vi "16.扫描引擎同步高阶 (Host).vi"() -> ()   [LabVIEW 2019]
uses:
  <vilib>/Platform/TimedLoop/XDataNode/wakeup.ctl
  <vilib>/Platform/TimedLoop/XDataNode/XDNodeRunTimeDep.lvlib
  <vilib>/Platform/TimedLoop/XDataNode/nitl_modes.ctl
  <vilib>/Platform/TimedLoop/XDataNode/timing_clust.ctl
  <vilib>/Platform/TimedLoop/XDataNode/XDataNode.xnode
  <vilib>/rvi/interface/nirviReadWriteControl/nirviReadWriteControl.xnode
  <vilib>/rvi/interface/Simulation/niFpgaSimulationCallBeginRW.vi
  <vilib>/rvi/errors/niLvFpgaAdjustHostInterfaceError.vi
  <vilib>/rvi/interface/nirviCloseFPGA/nirviCloseFPGA.xnode
  <vilib>/rvi/interface/nirviOpenFPGA/nirviOpenFPGA.xnode
  <vilib>/Platform/TimedLoop/XDataNode/loadnilvce.vi
  <vilib>/FPGAPlugInAG/ELVIS III/niLvFpga_Open_ELVIS III.vi
  <vilib>/rvi/interface/common/dynamic/niFpgaDynamicAddResources.vi
  NiFpgaLv.dll
  <vilib>/Utility/error.llb/Error Cluster From Error Code.vi
  <vilib>/FPGAPlugInAG/Dynamic/niLvFpga_Close_Dynamic.vi
panel:
  out "Error Out":errorcluster
  in  "Reset Missed Falling Edge Latch":bool
  out "Missed Falling Edge Instantaneous":bool
  out "Scan Clock High Time (FPGA clock ticks)":u32
  in  "Adjust FPGA Acquisition Delay\n**Watch for Missed Falling Edge**":u32(slide) scale=0.0..1000000.0
  out "Missed Falling Edge Latched":bool
  out "Host Loop Finished Late? [i-1]":bool
  in  "stop":bool
  out "Digital Waveform Data from FPGA":i16(graph)
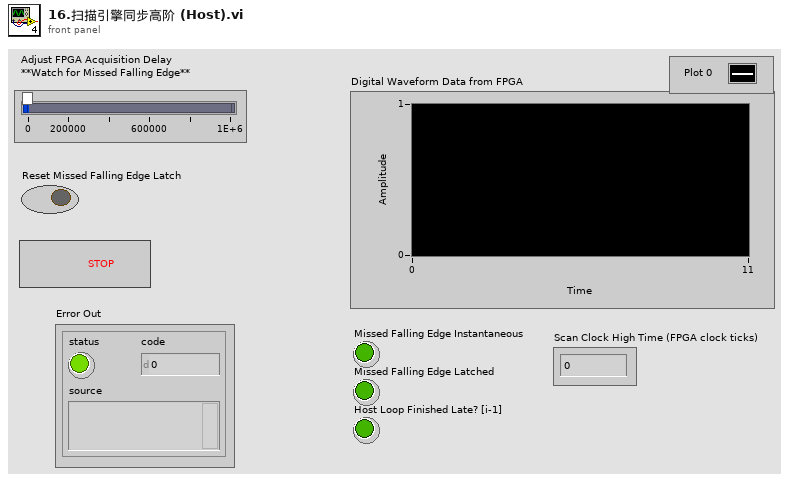
[diagram p1: front panel]
types:
  T1 = typedef "XDNodeRunTimeDep.lvlib/timing_clust.ctl" = cluster{"Expected End [f-1]":u64, "Actual End [f-1]":u64, "Finished Late? [f-1]":bool, "Expected End [i-1]":u64, "Actual End [i-1]":u64, "Finished Late? [i-1]":bool, "Expected Start [i]":u64, "Actual Start [i]":u64, "Expected Start [f]":u64, "Actual Start [f]":u64, "Source Name":string, "Structure Name":string, "Period":i64, "Deadline":i64, "Offset":i64, "Start":i64, "Priority":i32, "Timeout":i32, "Mode":T2, "Wakeup Reason":T3, "Error":errorcluster, "Source Type":string, "Secondary Source Type":string, "Global End Time":u64, "Global Start Time":u64, "Frame Duration":u64, "Iteration Duration":u64, "Assigned CPU":i32, "I/O Scan Engine Mode":u32}
  T2 = typedef "XDNodeRunTimeDep.lvlib/nitl_modes.ctl" = enum32{"No Change", "Process missed periods, maintain original phase", "Discard missed periods, maintain original phase", "Process missed periods, ignore original phase", "Discard missed periods, ignore original phase"}
  T3 = typedef "XDNodeRunTimeDep.lvlib/wakeup.ctl" = enum32{"Normal", "Aborted", "Asynchronous wakeup", "Timing source error", "Timed loop error", "Timeout"}
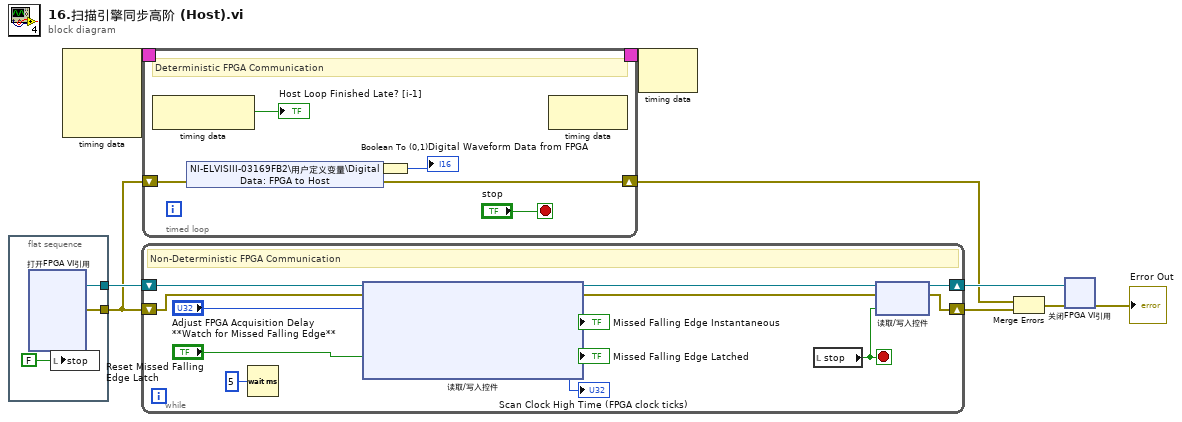
[diagram p0: block diagram]
diagram:
  n1 = flat-sequence {
    tunnel: [w12] -> w7
    tunnel: [w11] -> w6
    frame #0 {
      n2 = xnode "打开FPGA VI引用"() -> ("FPGA VI引用输出"=w12:refnum<k20>, "错误输出"=w11:errorcluster)  [unwired: 2 in]
      n3 = local write "stop"(FALSE ("stop")) -> ()
    }
  }
  n4 = node-c288() -> (w9:T1)  [unwired: 4 in]
  n5 = while {
    shift-right: [w22] -> w3
    shift-left: w6 -> [w23]
    shift-right: [w21] -> w5
    shift-left: w7 -> [w25]
    stop <- w24 stop-if-true
    # "Non-Deterministic FPGA Communication"
    n6 = Wait (ms)(milliseconds to wait=u32 5) -> ()  [unwired: 1 out]
    n7 = xnode "读取/写入控件"("FPGA VI引用输入"=w25, "错误输入"=w23, "Delay Time"="Adjust FPGA Acquisition Delay\n**Watch for Missed Falling Edge**", "Reset Missed Falling Edge Latch"="Reset Missed Falling Edge Latch") -> ("FPGA VI引用输出"=w14:refnum<k20>, "错误输出"=w13:errorcluster, "Missed Falling Edge Instantaneous"=→"Missed Falling Edge Instantaneous":bool, "Missed Falling Edge Latched"=→"Missed Falling Edge Latched":bool, "Scan Clock High Time"=→"Scan Clock High Time (FPGA clock ticks)":u32)
    n8 = local read "stop"() -> (w24:bool)
    n9 = xnode "读取/写入控件"("FPGA VI引用输入"=w14, "错误输入"=w13, "Stop"=w24) -> ("FPGA VI引用输出"=w21:refnum<k20>, "错误输出"=w22:errorcluster)
  }
  n10 = timed-loop {
    timing: w9 -> [_]
    timing-out: [_] -> w8
    shift-right: [w26] -> w2
    shift-left: w6 -> [w27]
    stop <- "stop" stop-if-true
    # "Deterministic FPGA Communication"
    n11 = node-c288() -> (→"Host Loop Finished Late? [i-1]":bool)  [unwired: 1 in]
    n12 = shared-variable "NI-ELVISIII-03169FB2\\用户定义变量\\Digital Data: FPGA to Host"(error in=w27) -> (w28:bool, error out=w26:errorcluster)
    n13 = Boolean To (0,1)(Boolean=w28) -> (0, 1=→"Digital Waveform Data from FPGA":i16)
    n14 = node-c288() -> ()  [unwired: 1 in, 1 out]
  }
  n15 = node-c288(w8) -> ()  [unwired: 1 out]
  n16 = Merge Errors(w2, w3) -> (w4:errorcluster)
  n17 = xnode "关闭FPGA VI引用"("FPGA VI引用输入"=w5, "错误输入"=w4) -> ("错误输出"=→"Error Out":errorcluster)
